vi "PH_Switch.constructor.vi"(0 "name":string, 2 "data in":string, 5 "error in(no error)":errorcluster) -> (14 "i ref out":refnum<vi>, 16 "data out":string, 19 "error out":errorcluster)   [LabVIEW 2014, in "PH_Switch.lvlib"]
doc: "This class is forseen to control easy switches with up to two end position sensors using Beckhoff.\n\nThis class is part of the PHELIX device layer.\n\nauthor: Stefan Götte, GSI\n\nLicense Agreement for this software:\n\nCopyright (C)\nGesellschaft für Schwerionenforschung, GSI\nPlanckstr. 1\n64291 Darmstadt\nGermany\n\nContact: D.Beck@gsi.de \n\nThis program is free software; you can redistribute it and/or modify it under the terms of the \nGNU General Public License as published by the Free Software Foundation; either version 2 of \nthe license, or (at your option) any later version.\n\nThis program is distributed in the hope that it will be useful, but WITHOUT ANY WARRANTY; \nwithout even the implied warranty of MERCHANTABILITY or FITNESS FOR A PARTICULAR PURPOSE. See the GNU General License for more details (http://www.gnu.org).\n\nGesellschaft für Schwerionenforschung, GSI\nPlanckstr. 1, 64291 Darmstadt, Germany\nFor all questions and ideas contact: M.Richter@gsi.de, H.Brand@gsi.de or D.Beck@gsi.de.\nLast update: 16-JUN-2004"
uses:
  PH_Switch.lvlib
  CSCore/CSSystem/CSSystemLib/CSSystemLib.lvlib
  PH_Class/PH_Class.lvlib
  PH_PSDBWriter/PH_PSDBWriter.lvlib
  PH_StatusHandler/PH_StatusHandler.lvlib
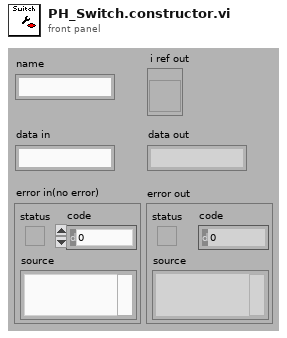
[diagram p1: front panel]
types:
  T1 = enum16{"SetAttribute", "GetAttribute", "CreateAttribute", "DestroyAttribute", "DestroyAllAtributes"}
  T2 = typedef "PH_Switch.lvlib/PH_Switch.i attribute.ctl" = cluster{"GUI Refs":T3, "Status true":T4, "Status false":T4, "Status Switch State":T4, "remote controlled":bool, "Tagname":cluster{"Switch":string, "True":string, "False":string}, "Beckhoff Instance":string, "Caption":cluster{"True":string, "False":string}, "Default State":string}
  T3 = typedef "PH_Switch.lvlib/PH_Switch.GUI Refs.ctl" = cluster{"true":refnum<vi>, "false":refnum<vi>, "Switch_state":refnum<vi>, "GUI-Knob":refnum<vi>, "Delete":refnum<vi>, "Function Textfield":refnum<vi>}
  T4 = typedef "PH_StatusHandler.lvlib/PH_StatusHandler.Status.ctl" = i16
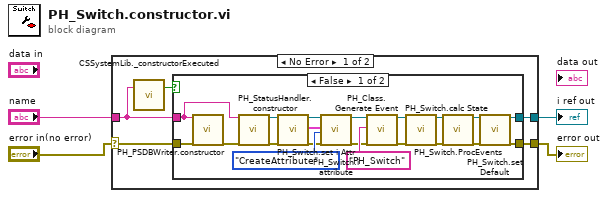
[diagram p0: block diagram]
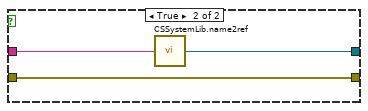
[diagram p2: hidden frame]
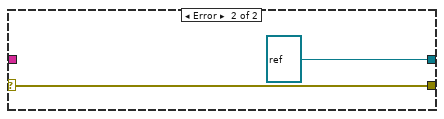
[diagram p3: hidden frame]
diagram:
  n1 = case shown="No Error" "error in(no error)" {
    selector: "error in(no error)" -> [w9 w34]
    tunnel: [w8 refnum<vi> refnum ("i ref out")] -> w4
    tunnel: [w7 w34] -> w3
    tunnel: "name" -> [w6 _]
    frame No Error {
      n2 = call "CSSystemLib._constructorExecuted.vi"("name"=w6) -> ("constructor executed?"=w5:bool)  [unwired: 18 in]
      n3 = case shown="False" w5 {
        tunnel: w9 -> [w14 w30]
        tunnel: [w29 w31] -> w8
        tunnel: [w28 w30] -> w7
        tunnel: w6 -> [w10 w32]
        frame False {
          n4 = call "PH_PSDBWriter.constructor.vi"("name"=w10, "error in"=w14) -> ("error out"=w12:errorcluster)  [unwired: 15 in, 2 out]
          n5 = call "PH_StatusHandler.constructor.vi"("name"=w10, "error in(no error)"=w12) -> ("i ref out"=w13:refnum<vi>, "error out"=w11:errorcluster)  [unwired: 15 in, 1 out]
          n6 = call "PH_Switch.set i Attr.vi"("VI in"=w13, "error in (no error)"=w11) -> ("VI out"=w26:refnum<vi>, "i Attribute"=w24:T2, "error out"=w25:errorcluster)  [unwired: 15 in]
          n7 = call "PH_Switch.i attribute.vi"("VI Refnum"=w26, "CLASS.i attribute"=w24, "Action"=T1."CreateAttribute", "error in (no error)"=w25) -> ("VI Refnum out"=w21:refnum<vi>, "error out"=w22:errorcluster)  [unwired: 13 in, 1 out]
          n8 = call "PH_Class.Generate Event.vi"("i ref in"=w21, "Class"="PH_Switch" ("event data"), "error in (no error)"=w22) -> ("i ref out"=w20:refnum<vi>, "error out"=w19:errorcluster)  [unwired: 15 in]
          n9 = call "PH_Switch.calc State.vi"("i ref in"=w20, "error in (no error)"=w19) -> ("i ref out"=w15:refnum<vi>, "error out"=w16:errorcluster)  [unwired: 16 in]
          n10 = call "PH_Switch.ProcEvents.vi"("i ref in"=w15, "error in (no error)"=w16) -> ("i ref out"=w17:refnum<vi>, "error out"=w18:errorcluster)  [unwired: 16 in]
          n11 = call "PH_Switch.set Default.vi"("i ref in"=w17, "error in"=w18) -> ("i ref out"=w29:refnum<vi>, "error out"=w28:errorcluster)  [unwired: 16 in]
        }
        frame True {
          n12 = call "CSSystemLib.name2ref.vi"("name"=w32) -> ("obj refnum"=w31:refnum<vi>)
        }
      }
    }
    frame Error {
    }
  }
  "i ref out" <- w4
  "error out" <- w3
